vi "Color Sensor(SubVI).vi"(0 "color_din":dbl) -> (4 "color_dout":dbl)   [LabVIEW 2017]
uses:
  <vilib>/functionblocks/Edge Detection/Edge Detect/Edge Detect.vi
  <vilib>/functionblocks/FB Core/FB Core.xnode
  <vilib>/functionblocks/NI_FunctionBlock Libraries.lvlib
panel:
  out "in":bool
  out "res":bool
  out "Waveform Chart":dbl(graph)
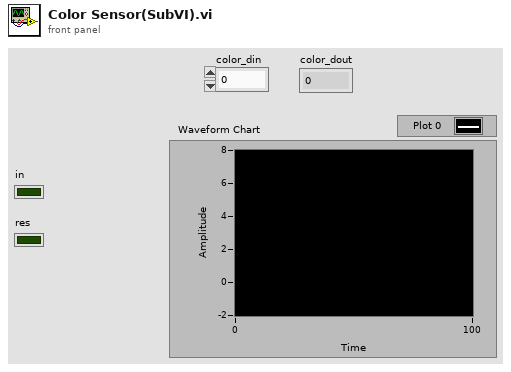
[diagram p1: front panel]
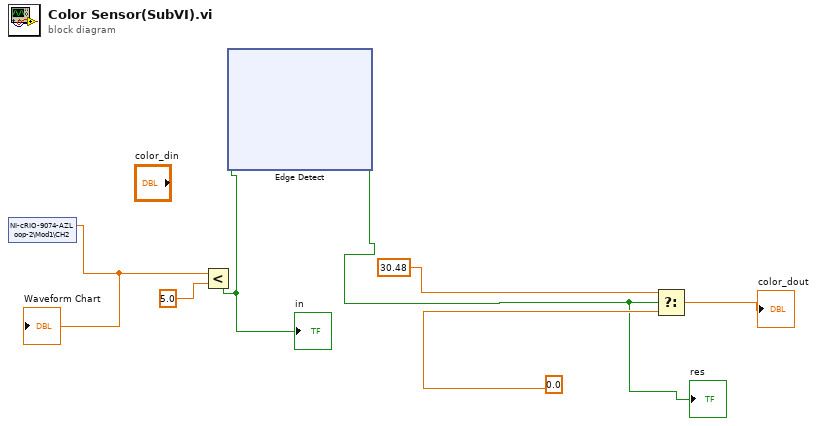
[diagram p0: block diagram]
diagram:
  n1 = shared-variable "NI-cRIO-9074-AZLoop-2\\Mod1\\CH2"() -> (w3:dbl)  [unwired: 1 in, 1 out]
  "Waveform Chart" <- w3
  n2 = Less?(x=w3, y=5.0) -> (x < y?=w1:bool)
  "in" <- w1
  n3 = xnode "Edge Detect"("input 1"=w1) -> ("output"=w2:bool)  [unwired: 2 in, 1 out]
  "res" <- w2
  n4 = Select(t=30.48, s=w2, f=0.0) -> (s? t:f=→"color_dout":dbl)
